vi "Teleop2.vi"(10 "Match Info":T1={"Autonomous Elapsed Seconds"=0.0, "TeleOp Elapsed Seconds"=0.0, "Disabled Elapsed Seconds"=0.0, "Visited Autonomous"=FALSE, "Visited TeleOp"=FALSE, "Visited Disabled"=FALSE, "Autonomous Settings"={"Autonomous Style"=enum."Independent", "VI Refnum"=refnum}}, 11 "Call Context":T2) -> ()   [LabVIEW 2018]
doc: "This VI is called for each TeleOp packet received from the DS where the robot is not disabled. It is often used to read from the joysticks and update I/O or to update setpoints for timed control loops. It should complete and return within 20 milliseconds or it may miss DS packets."
uses:
  <vilib>/Rock Robotics/WPI/DriverStation/WPI_DriverStationDerivedRobotMode.ctl
  <vilib>/Rock Robotics/WPI/DriverStation/WPI_DriverStationMatch Info.ctl
  <vilib>/Rock Robotics/WPI/ThirdParty/Phoenix-LabVIEW/Motor Controller/Controls/CTRE_Phoenix_MotorControl_ControlMode.ctl
  <vilib>/Rock Robotics/WPI/Utilities/WPI_GetSetVariantRefNum.vi
  <vilib>/Rock Robotics/WPI/ThirdParty/Phoenix-LabVIEW/Motor Controller/Get/CTRE_Phoenix_MotorController_GetVoltage.vi
  <vilib>/Rock Robotics/WPI/ThirdParty/Phoenix-LabVIEW/Motor Controller/Get/CTRE_Phoenix_MotorController_GetSelectedSensorData.vi
panel:
  out "SensorPos (rotations)":i32
  out "Target Position (rotations)":dbl
  out "SensorRPM Velocity Raw":i32
  in  "I Zone":dbl
  in  "F - Generally is zero for position-servo":dbl
  in  "D":dbl
  in  "I":dbl
  in  "P":dbl
  out "Applied Output":dbl
  out "Position Closed Loop Plots":cluster{dbl, "Position (Raw Sensor Units)":i32}(graph)
  # "Press and Hold Button1 to drive Talon directly.  Make sure sensor position moves in positive direction when Talon LEDs are green.\n\nMomentary press Button2 to activate Position closed-loop.  The gamepad y-axis is sampled once and scaled to provide a target set point.\n\nPress Button3 to \"zero\" the sensor position.\n\nPress Button4 to \"seed\" the Sensor position with the Absolute Position reported by the CTRE Magnetic Encoder."
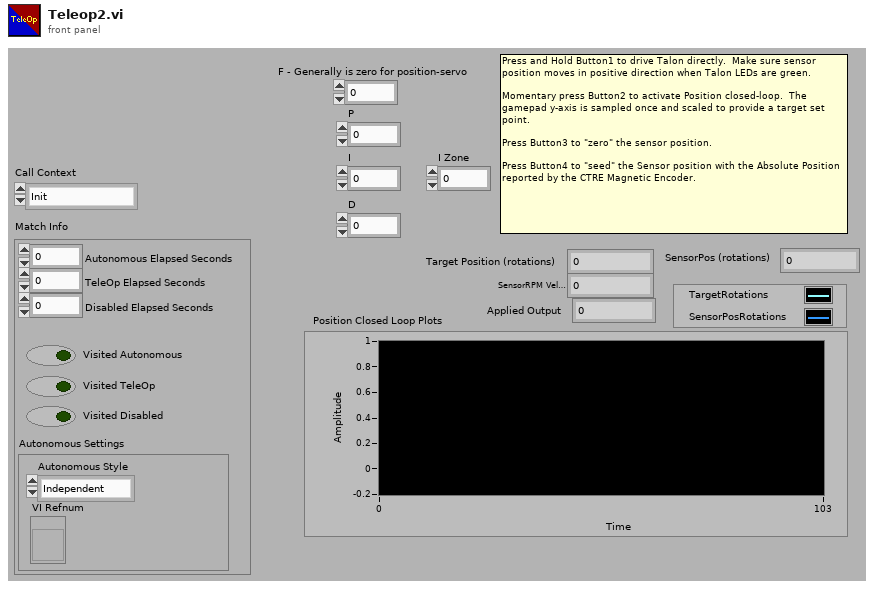
[diagram p1: front panel]
types:
  T1 = typedef "WPI_DriverStationMatch Info.ctl" = cluster{"Autonomous Elapsed Seconds":dbl, "TeleOp Elapsed Seconds":dbl, "Disabled Elapsed Seconds":dbl, "Visited Autonomous":bool, "Visited TeleOp":bool, "Visited Disabled":bool, "Autonomous Settings":cluster{"Autonomous Style":enum16{"Iterative", "Independent"}, "VI Refnum":refnum<vi>}}
  T2 = typedef "WPI_DriverStationDerivedRobotMode.ctl" = enum16{"Init", "Execute", "Stop"}
  T3 = typedef "WPI_JoystickDevRef.ctl" = cluster{"Device":T4}
  T4 = typedef "WPI_JoystickDeviceEnum.ctl" = enum16{"USB 0", "USB 1", "USB 2", "USB 3", "USB 4", "USB 5"}
  T5 = typedef "WPI_MotorControlDeviceRef.ctl" = cluster{"DeviceStatus":errorcluster, "Type":T6, "PWM":cluster{"PWM Channel":T7, "DeadBand":T8}, "CAN":cluster{"Device Number":u8, "SetOutput VI Ref":variant, "GetOutput VI Ref":variant, "Enable VI Ref":variant, "Disable VI Ref":variant, "Data":variant}, "Invert":bool, "DIO PWM":cluster{"PWM \"Enable\" Channel":T7, "DIOChannel":T9, "PWM Rate":dbl}}
  T6 = typedef "WPI_MotorControlType.ctl" = enum16{"PWM", "CAN", "DIO PWM"}
  T7 = typedef "FPGA_DIOPWMChannel.ctl" = enum8{"PWM 0", "PWM 1", "PWM 2", "PWM 3", "PWM 4", "PWM 5", "PWM 6", "PWM 7", "PWM 8", "PWM 9", "PWM MXP 0", "PWM MXP 1", "PWM MXP 2", "PWM MXP 3", "PWM MXP 4", "PWM MXP 5", "PWM MXP 6", "PWM MXP 7", "PWM MXP 8", "PWM MXP 9", "Invalid"}
  T8 = typedef "WPI_PWMDeadband.ctl" = cluster{"Name":string, "maxPositivePwm":i32, "minPositivePwm":i32, "centerPwm":i32, "maxNegativePwm":i32, "minNegativePwm":i32, "angularRange":u16}
  T9 = typedef "FPGA_DIOChannel.ctl" = enum8{"DIO 0", "DIO 1", "DIO 2", "DIO 3", "DIO 4", "DIO 5", "DIO 6", "DIO 7", "DIO 8", "DIO 9", "DIO MXP 0", "DIO MXP 1", "DIO MXP 2", "DIO MXP 3", "DIO MXP 4", "DIO MXP 5", "DIO MXP 6", "DIO MXP 7", "DIO MXP 8", "DIO MXP 9", "DIO MXP 10", "DIO MXP 11", "DIO MXP 12", "DIO MXP 13", "DIO MXP 14", "DIO MXP 15", "SPI Port CS1", "SPI Port CS2", "SPI Port CS3", "SPI Port MISO", "SPI Port MOSI", "Invalid"}
  T10 = typedef "CTRE_Phoenix_MotorControl_ControlMode.ctl" = u16
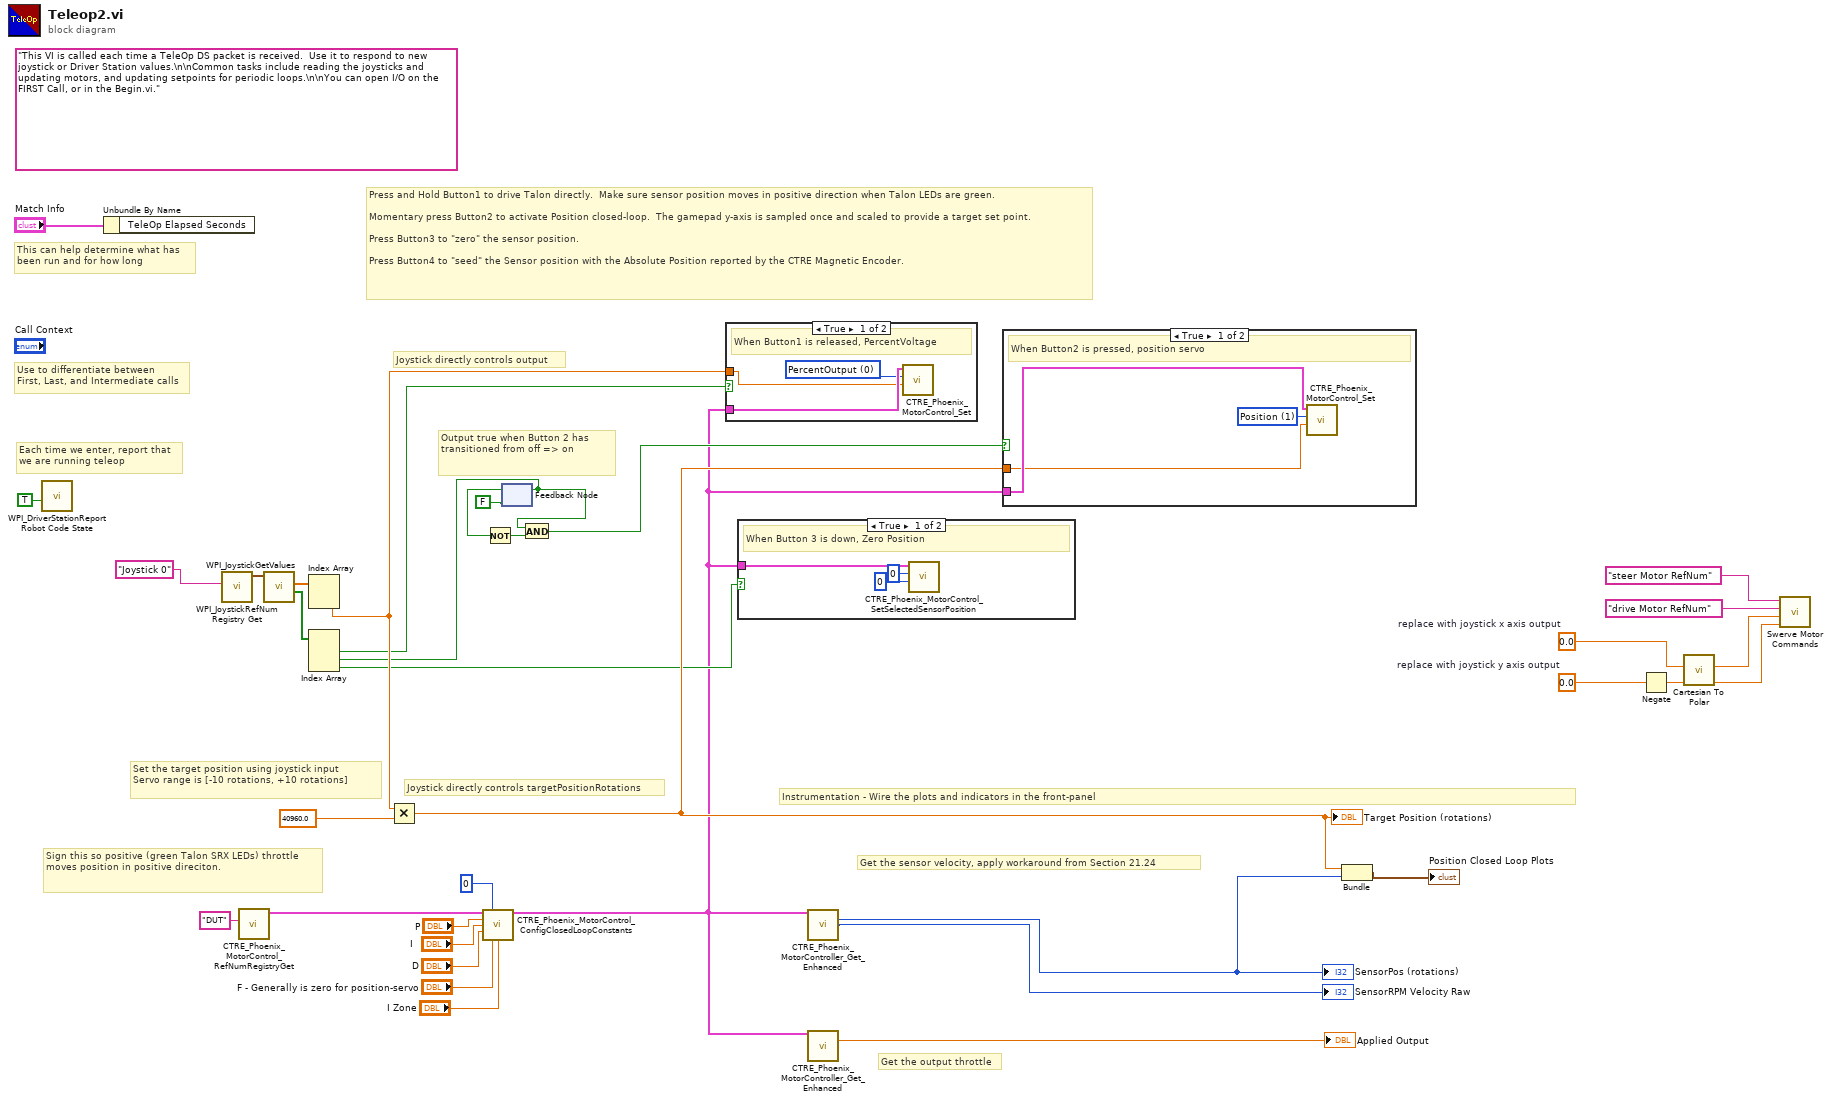
[diagram p0: block diagram]
diagram:
  w1 = 0.0  # replace with joystick y axis output
  w2 = 0.0  # replace with joystick x axis output
  (unwired) "This VI is called each time a TeleOp DS packet is received.  Use it to respond to new joystick or Driver Station values.\n\nCommon tasks include reading the joysticks and updating motors, and updating setpoints for periodic loops.\n\nYou can open I/O on the FIRST Call, or in the Begin.vi."
  # "Sign this so positive (green Talon SRX LEDs) throttle moves position in positive direciton."
  # "Instrumentation - Wire the plots and indicators in the front-panel"
  # "Output true when Button 2 has transitioned from off => on"
  # "Press and Hold Button1 to drive Talon directly.  Make sure sensor position moves in positive direction when Talon LEDs are green.\n\nMomentary press Button2 to activate Position closed-loop.  The gamepad y-axis is sampled once and scaled to provide a target set point.\n\nPress Button3 to \"zero\" the sensor position.\n\nPress Button4 to \"seed\" the Sensor position with the Absolute Position reported by the CTRE Magnetic Encoder."
  # "Get the output throttle"
  # "Get the sensor velocity, apply workaround from Section 21.24"
  # "Joystick directly controls targetPositionRotations"
  # "Joystick directly controls output"
  # "Set the target position using joystick input\nServo range is [-10 rotations, +10 rotations]"
  # "Each time we enter, report that\nwe are running teleop"
  # "Use to differentiate between\nFirst, Last, and Intermediate calls"
  # "This can help determine what has\nbeen run and for how long"
  n1 = call <vilib>:"WPI_DriverStationReport Robot Code State.vi"("TeleOp"=TRUE ("Autonomous")) -> ()  [unwired: 10 in, 1 out]
  n2 = Unbundle By Name("Match Info") -> ()  [unwired: 1 out]
  n3 = call <vilib>:"WPI_JoystickRefNum Registry Get.vi"("refnum name"="Joystick 0") -> ("JoystickDevRef"=w34:T3)  [unwired: 1 in, 9 out]
  n4 = call <vilib>:"CTRE_Phoenix_MotorControl_RefNumRegistryGet.vi"("refnum name"="DUT") -> ("PhoenixMotorControlDevRef"=w8:T5)  [unwired: 9 in, 1 out]
  n5 = call <vilib>:"WPI_JoystickGetValues.vi"("JoystickDevRef"=w34) -> ("Buttons"=w31:bool[], "Axes"=w32:dbl[])  [unwired: 6 in, 3 out]
  n6 = Index Array(array=w32) -> (element #2=w28:dbl)  [unwired: 2 in, 1 out]
  n7 = Index Array(array=w31) -> (element #1=w25:bool, element #2=w23:bool, element #3=w21:bool)  [unwired: 3 in]
  n8 = Multiply(x=w28, y=40960.0) -> (x*y=w22:dbl)
  "Target Position (rotations)" <- w22
  n9 = call <vilib>:"CTRE_Phoenix_MotorControl_ConfigClosedLoopConstants.vi"("PhoenixMotorControlDevRef"=w8, "slotIdx"=0, "P"="P", "I"="I", "D"="D", "F"="F - Generally is zero for position-servo", "I Zone"="I Zone") -> ("PhoenixMotorControlDevRef"=w11:T5)  [unwired: 7 in, 1 out]
  n10 = feedback-in #1(w23) -> ()
  n11 = feedback #1(FALSE) -> (w24:bool)
  n12 = Not(x=w24) -> (.not. x?=w26:bool)
  n13 = And(x=w23, y=w26) -> (x .and. y?=w20:bool)
  n14 = case shown="True" w25 {
    tunnel: w28 -> [w38 _]
    tunnel: w11 -> [w39 _]
    frame True {
      w37 = T10 0 items=["PercentOutput"=0, "Position"=1, "Velocity"=2, "Follower"=5, "MotionProfile"=6, "MotionMagic"=7, "MotionMagicArc"=8, "TimedPercentOutput"=9, "Disabled"=15] ("Control Mode")
      # "When Button1 is released, PercentVoltage"
      n15 = call <vilib>:"CTRE_Phoenix_MotorControl_Set.vi"("Output"=w38, "Control Mode"=w37, "PhoenixMotorControlDevRef"=w39) -> ()  [unwired: 7 in, 2 out]
    }
    frame False {
    }
  }
  n16 = case shown="True" w21 {
    tunnel: w11 -> [w42 _]
    frame True {
      # "When Button 3 is down, Zero Position"
      n17 = call <vilib>:"CTRE_Phoenix_MotorControl_SetSelectedSensorPosition.vi"("pidLoopIdx"=u32 0, "New Sensor Position"=0, "PhoenixMotorControlDevRef"=w42) -> ()  [unwired: 7 in, 2 out]
    }
    frame False {
    }
  }
  n18 = call-poly <vilib>:"CTRE_Phoenix_MotorController_Get_Enhanced.vi"("PhoenixMotorControlDevRef"=w11) -> ("Position (Raw Sensor Units)"=w12:i32, "Velocity (Raw Sensor Units per 100 ms)"=→"SensorRPM Velocity Raw":i32)  [unwired: 11 in, 2 out]
  "SensorPos (rotations)" <- w12
  n19 = call-poly <vilib>:"CTRE_Phoenix_MotorController_Get_Enhanced.vi"("PhoenixMotorControlDevRef"=w11) -> ("Percent Output"=→"Applied Output":dbl)  [unwired: 10 in, 4 out]
  n20 = case shown="True" w20 {
    tunnel: w22 -> [w44 _]
    tunnel: w11 -> [w45 _]
    frame True {
      w43 = T10 1 items=["PercentOutput"=0, "Position"=1, "Velocity"=2, "Follower"=5, "MotionProfile"=6, "MotionMagic"=7, "MotionMagicArc"=8, "TimedPercentOutput"=9, "Disabled"=15] ("Control Mode")
      # "When Button2 is pressed, position servo"
      n21 = call <vilib>:"CTRE_Phoenix_MotorControl_Set.vi"("Output"=w44, "Control Mode"=w43, "PhoenixMotorControlDevRef"=w45) -> ()  [unwired: 7 in, 2 out]
    }
    frame False {
    }
  }
  n22 = Bundle(w22, "Position (Raw Sensor Units)"=w12) -> (→"Position Closed Loop Plots":cluster{dbl, "Position (Raw Sensor Units)":i32})  [unwired: 1 in]
  n23 = Negate(x=w1) -> (-x=w3:dbl)
  n24 = call "Cartesian To Polar.vi"("Joystick y axis input"=w3, "Joystick x axis input"=w2) -> ("Theta (deg)"=w4:dbl, "Magnitude"=w5:dbl)  [unwired: 8 in]
  n25 = call "Swerve Motor Commands.vi"("Steer motor reference name"="steer Motor RefNum", "Drive motor reference name"="drive Motor RefNum", "Speed command"=w5, "Direction command (deg)"=w4) -> ()  [unwired: 6 in]
